vi "Utility Read From Register.vi"(6 "Direct Action?":bool, 7 "Unit Address (1)":u8=1, 8 "error in (no error)":errorcluster, 9 "Num Of Reg (1)":u16=1 min=1 step=1, 10 "Register Address (0)":u16, 11 "VISA resource name":refnum<visa-resource-name>) -> (0 "error out":errorcluster, 2 "Data":i16[](array[numeric]), 3 "VISA resource name out":refnum<visa-resource-name>)   [LabVIEW 2010]
doc: "This VI reads value from specified registers of specified unit."
uses:
  MBDRV_Command Data.ctl
  MBDRV_Action.ctl
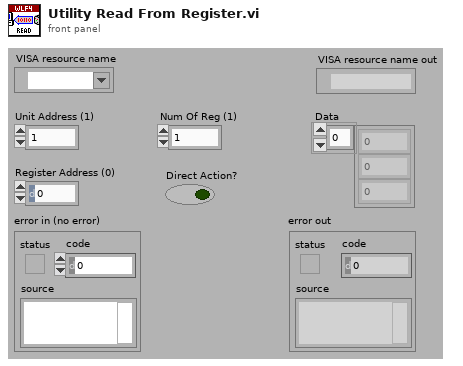
[diagram p1: front panel]
types:
  T1 = typedef "MBDRV_Command Data.ctl" = cluster{"Action":T2, "Com Port":string, "Register Address":u16, "Data To Write/Num To Read":i16}
  T2 = typedef "MBDRV_Action.ctl" = enum16{"Write", "Read"}
  T3 = enum16{"By The Number of Bytes", "Copy Of the Sent Message"}
  T4 = typedef "MBDRV_Response List.ctl" = T5[]
  T5 = typedef "MBDRV_Response.ctl" = cluster{"Action":T2, "Com Port":string, "Register Address":u16, "Data":i16[]}
  T6 = cluster{"Read Buffer[0]":u8, "Read Buffer[1]":u8}
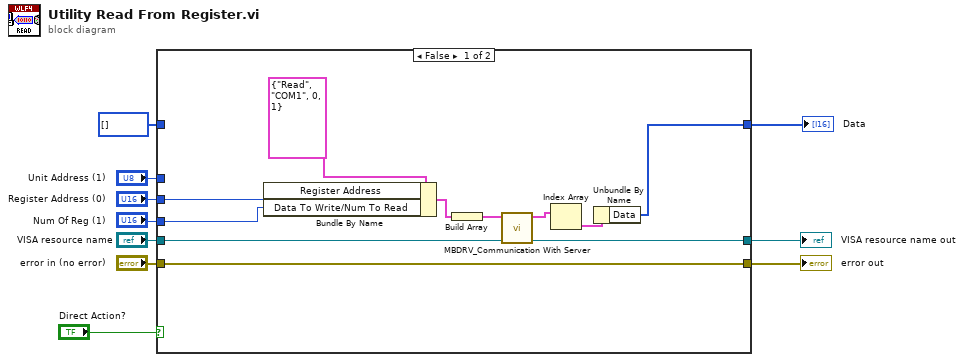
[diagram p0: block diagram]
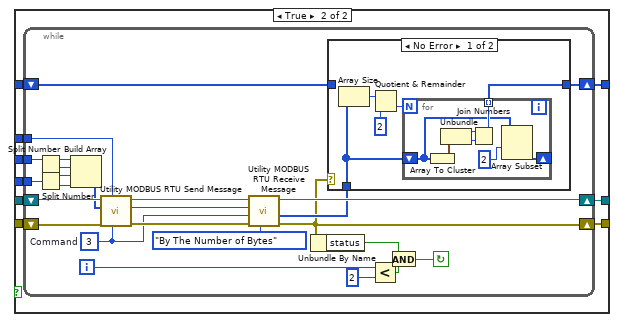
[diagram p2: hidden frame]
diagram:
  n1 = case shown="False" "Direct Action?" {
    tunnel: "VISA resource name" -> [w20 w29]
    tunnel: [w20 w28] -> w9
    tunnel: "Num Of Reg (1)" -> [w16 w27]
    tunnel: [w11 w26] -> w7
    tunnel: u16[] [] -> [_ w25]
    tunnel: "error in (no error)" -> [w19 w24]
    tunnel: [w19 w23] -> w4
    tunnel: "Register Address (0)" -> [w17 w22]
    tunnel: "Unit Address (1)" -> [_ w21]
    frame False {
      n2 = Bundle By Name(cluster=T1 {"Action"=enum."Read", "Com Port"="COM1", "Register Address"=0, "Data To Write/Num To Read"=1} ("Command"), "Register Address"=w17, "Data To Write/Num To Read"=w16) -> (w15:T1)
      n3 = Build Array(w15) -> (w14:T1[])
      n4 = call "MBDRV_Communication With Server.vi"("Write To PLC"=w14) -> ("Read From PLC"=w13:T4)  [unwired: 9 in, 1 out]
      n5 = Index Array(array=w13) -> (element=w12:T5)  [unwired: 1 in]
      n6 = Unbundle By Name(w12) -> ("Data"=w11:i16[])
    }
    frame True {
      n7 = while {
        tunnel: w21 -> [w33]
        shift-right: [w51] -> w28
        shift-left: w29 -> [w52]
        tunnel: w22 -> [w41]
        tunnel: w27 -> [w37]
        shift-right: [w39] -> w26
        shift-left: w25 -> [w38]
        shift-right: [w31] -> w23
        shift-left: w24 -> [w30]
        i -> [w47]
        stop <- w49 continue-if-true
        w48 = u8 3  # Command
        n8 = Split Number(x=w41) -> (hi(x)=w43:u8, lo(x)=w42:u8)
        n9 = Split Number(x=w37) -> (hi(x)=w36:u8, lo(x)=w35:u8)
        n10 = Build Array(w43, w42, w36, w35) -> (w44:u8[])
        n11 = call "Utility MODBUS RTU Send Message.vi"("Command (0)"=w48, "Unit Address (1)"=w33, "error in (no error)"=w30, "Message (empty array)"=w44, "VISA resource name"=w52) -> ("error out"=w54:errorcluster, "Length Of Sent MSG"=w34:u8, "VISA resource name out"=w53:refnum<visa-resource-name>)  [unwired: 4 in]
        n12 = call "Utility MODBUS RTU Receive Message.vi"("Receive Message Type (0: By The Number Of Bytes)"=T3."By The Number of Bytes" ("Receive Message Type"), "error in (no error)"=w54, "Sent Command (0)"=w48, "Length Of Sent MSG (0)"=w34, "VISA resource name"=w53) -> ("error out"=w31:errorcluster, "Read Buffer"=w40:u8[], "VISA resource name out"=w51:refnum<visa-resource-name>)  [unwired: 4 in]
        n13 = Unbundle By Name(w31) -> ("status"=w50:bool)
        n14 = case shown="No Error" w31 {
          tunnel: w40 -> [w59 _]
          tunnel: [w58 w67] -> w39
          tunnel: w38 -> [_ w67]
          frame No Error {
            n15 = Array Size(array=w59) -> (size(s)=w57:i32)
            n16 = Quotient & Remainder(x=w57, y=2) -> (floor(x/y)=w55:i32)  [unwired: 1 out]
            n17 = for {
              N: w55 -> [_]
              shift-right: [w61] -> _
              shift-left: w59 -> [w62]
              tunnel: [w63] -> w58 mode=indexing
              n18 = Array To Cluster(array=w62) -> (cluster=w66:T6)
              n19 = Unbundle(w66) -> ("Read Buffer[0]"=w64:u8, "Read Buffer[1]"=w65:u8)
              n20 = Join Numbers(hi=w64, lo=w65) -> ((hi.lo)=w63:u16)
              n21 = Array Subset(array=w62, index=2) -> (w61:u8[])  [unwired: 1 in]
            }
          }
          frame Error {
          }
        }
        n22 = Less?(x=w47, y=2) -> (x < y?=w46:bool)
        n23 = And(x=w50, y=w46) -> (x .and. y?=w49:bool)
      }
    }
  }
  "error out" <- w4
  "VISA resource name out" <- w9
  "Data" <- w7
